vi "转换ROI对比.vi"() -> ()   [LabVIEW 2018]
uses:
  <vilib>/vision/NI_Vision_Development_Module.lvlib
panel:
  out "Image 2":T1(plugin-control)
  out "error out":errorcluster
  out "元素":T2 {"Contours"."Type" items=["No Selection", "Point", "Line", "Rectangle", "Oval", "Polygon", "Freehand Region", "Annulus", "Unused2", "Unused3", "Broken Line", "Freehand Line", "Rotated Rectangle"]}
  in  "索引":i32
  out "Image":T1(plugin-control)
  in  "路径":path
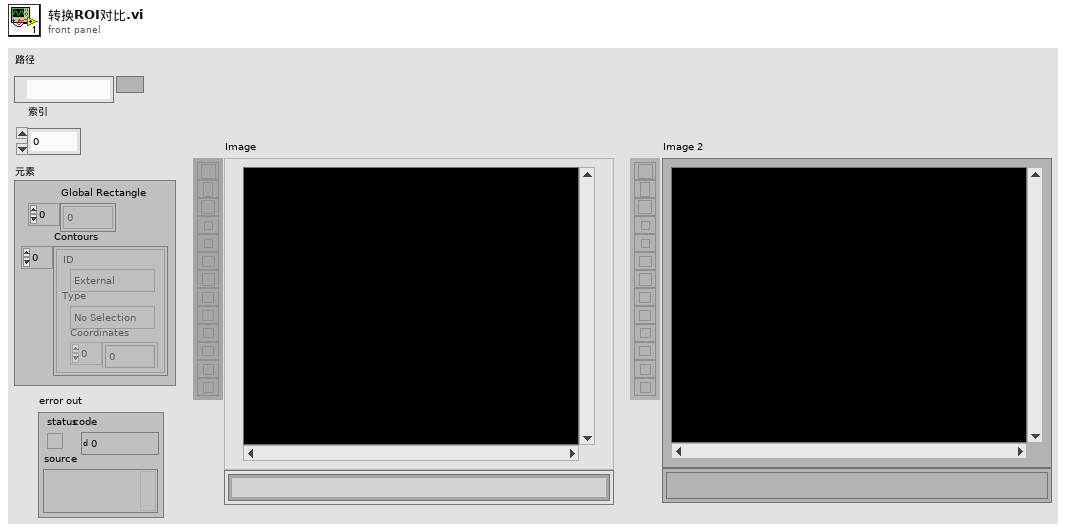
[diagram p1: front panel]
types:
  T1 = typedef "IMAQ Image.ctl" = refnum<image>
  T2 = typedef "ROI Descriptor" = cluster{"Global Rectangle":i32[], "Contours":cluster{"ID":enum32{"External", "Internal"}, "Type":u32, "Coordinates":i32[]}[]}
  T3 = typedef "Image Type" = u32
  T4 = cluster{"ID":enum32{"External", "Internal"}, "Type":u32, "Coordinates":i32[]}[]
  T5 = cluster{"ID":enum32{"External", "Internal"}, "Type":u32, "Coordinates":i32[]}
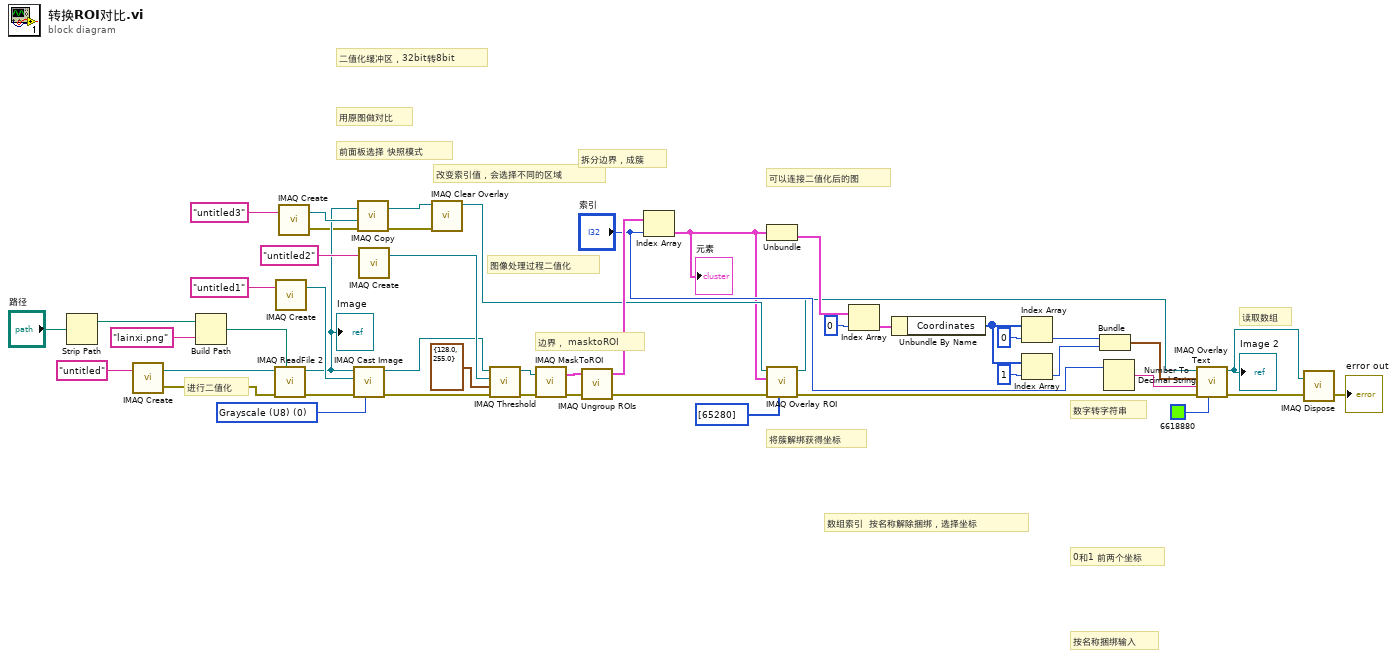
[diagram p0: block diagram]
diagram:
  w39 = T3 0 items=["Grayscale (U8)", "Grayscale (I16)", "Grayscale (SGL)", "Complex (CSG)", "RGB (U32)", "HSL (U32)", "RGB (U64)", "Grayscale (U16)"] ("Image Type")
  # "改变索引值，会选择不同的区域"
  # "前面板选择 快照模式"
  # "按名称捆绑输入"
  # "读取数组"
  # "0和1 前两个坐标"
  # "数组索引  按名称解除捆绑，选择坐标"
  # "将簇解绑获得坐标"
  # "数字转字符串"
  # "可以连接二值化后的图"
  # "用原图做对比"
  # "拆分边界，成簇"
  # "边界， masktoROI"
  # "图像处理过程二值化"
  # "二值化缓冲区，32bit转8bit"
  # "进行二值化"
  n1 = Strip Path(path="路径") -> (stripped path=w47:path)  [unwired: 1 out]
  n2 = call "IMAQ Create"("Image Name"="untitled") -> ("New Image"=w44:T1, "error out"=w43:errorcluster)  [unwired: 4 in]
  n3 = Build Path(base path=w47, name or relative path="lainxi.png" ("名称或相对路径")) -> (appended path=w45:path)
  n4 = call "IMAQ ReadFile 2"("File Path"=w45, "error in (no error)"=w43, "Image"=w44) -> ("error out"=w38:errorcluster, "Image Out"=w25:T1)  [unwired: 4 in, 3 out]
  "Image" <- w25
  n5 = call "IMAQ Create"("Image Name"="untitled1") -> ("New Image"=w40:T1)  [unwired: 4 in, 1 out]
  n6 = call "IMAQ Create"("Image Name"="untitled3") -> ("New Image"=w26:T1, "error out"=w24:errorcluster)  [unwired: 4 in]
  n7 = call "IMAQ Cast Image"("Image Type"=w39, "error in (no error)"=w38, "Image Dst"=w40, "Image Src"=w25) -> ("error out"=w34:errorcluster, "Image Dst Out"=w36:T1)  [unwired: 6 in]
  n8 = call "IMAQ Copy"("error in (no error)"=w24, "Image Dst"=w26, "Image Src"=w25) -> ("error out"=w22:errorcluster, "Image Dst Out"=w23:T1)  [unwired: 3 in]
  n9 = call "IMAQ Create"("Image Name"="untitled2") -> ("New Image"=w37:T1)  [unwired: 4 in, 1 out]
  n10 = call "IMAQ Clear Overlay"("error in (no error)"=w22, "Image"=w23) -> ("Image Out"=w21:T1)  [unwired: 8 in, 1 out]
  n11 = call "IMAQ Threshold"("error in (no error)"=w34, "Range"=cluster{"Lower value":sgl, "Upper value":sgl} {"Lower value"=128.0, "Upper value"=255.0}, "Image Dst"=w37, "Image Src"=w36) -> ("error out"=w32:errorcluster, "Image Dst Out"=w20:T1)  [unwired: 6 in]
  n12 = call "IMAQ MaskToROI"("Image"=w20, "error in (no error)"=w32) -> ("ROI Descriptor"=w31:T2, "error out"=w30:errorcluster)  [unwired: 5 in, 1 out]
  n13 = call "IMAQ Ungroup ROIs"("error in (no error)"=w30, "ROI Descriptor"=w31) -> ("error out"=w28:errorcluster, "ROI Descriptors out"=w29:T2[])  [unwired: 2 in]
  n14 = Index Array(array=w29, index="索引") -> (element=w18:T2)
  "元素" <- w18
  n15 = Unbundle(w18) -> ("Contours"=w17:T4)  [unwired: 1 out]
  n16 = call "IMAQ Overlay ROI"("Colors (Green)"=u32[] [65280], "error in (no error)"=w28, "ROI Descriptor"=w18, "Image"=w21) -> ("error out"=w7:errorcluster, "Image Out"=w6:T1)  [unwired: 6 in]
  n17 = Index Array(array=w17, index=0 ("索引")) -> (element=w15:T5)
  n18 = Unbundle By Name(w15) -> ("Coordinates"=w12:i32[])
  n19 = Index Array(array=w12, index=0 ("索引")) -> (element=w11:i32)
  n20 = Index Array(array=w12, index=1 ("索引")) -> (element=w10:i32)
  n21 = Bundle(w11, w10) -> (w9:cluster{i32, i32})  [unwired: 1 in]
  n22 = Number To Decimal String(number="索引") -> (decimal integer string=w8:string)  [unwired: 1 in]
  n23 = call "IMAQ Overlay Text"("Text Color (black)"=u32 6618880, "error in (no error)"=w7, "String"=w8, "Origin"=w9, "Image"=w6) -> ("error out"=w5:errorcluster, "Image Out"=w3:T1)  [unwired: 5 in]
  "Image 2" <- w3
  n24 = call "IMAQ Dispose"("Image"=w3, "error in (no error)"=w5) -> ("error out"=→"error out":errorcluster)  [unwired: 4 in]
